vi "Bytes to word.vi"(7 "Index":i32, 8 "Image Data in":u8[](array[numeric])) -> (1 "Index+2":i32, 2 "Word":u16)   [LabVIEW 2014, in "LAVA TIFF File Reader.lvlib"]
uses:
  LAVA TIFF File Reader.lvlib
  Globals.vi
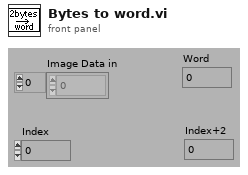
[diagram p1: front panel]
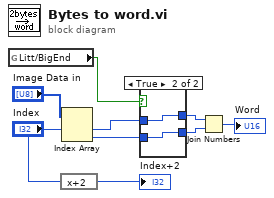
[diagram p0: block diagram]
diagram:
  n1 = global read "Globals.vi" "Litt/BigEnd"() -> (w5:bool)
  n2 = expression code="x+2"("Index") -> (→"Index+2":i32)
  n3 = Index Array(array="Image Data in", index #1="Index") -> (element #1=w4:u8, element #2=w3:u8)  [unwired: 1 in]
  n4 = case shown="True" w5 {
    tunnel: w4 -> [w10 w13]
    tunnel: [w11 w13] -> w1
    tunnel: w3 -> [w11 w12]
    tunnel: [w10 w12] -> w2
    frame False {
    }
    frame True {
    }
  }
  n5 = Join Numbers(hi=w1, lo=w2) -> ((hi.lo)=→"Word":u16)
